vi "Locate Section.vi"(8 "error in":errorcluster, 10 "section":string, 11 "key lookup":variant) -> (0 "error out":errorcluster, 1 "Section Definition":T1, 2 "found?":bool, 3 "key lookup out":variant)   [LabVIEW 2012, in "configlib.lvlib"]
uses:
  configlib.lvlib
  Section Definition.ctl
  File Section.ctl
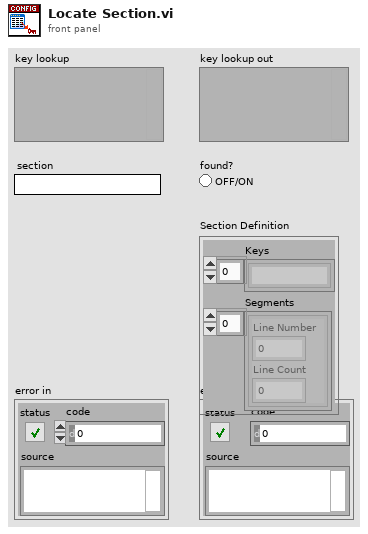
[diagram p1: front panel]
types:
  T1 = typedef "configlib.lvlib/Section Definition.ctl" = cluster{"Keys":string[], "Segments":T2[]}
  T2 = typedef "configlib.lvlib/File Section.ctl" = cluster{"Line Number":i32, "Line Count":i32}
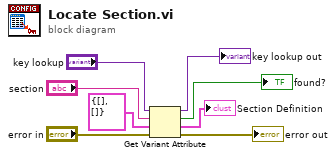
[diagram p0: block diagram]
diagram:
  n1 = Get Variant Attribute(Variant="key lookup", name="section", default value (empty Variant)=T1 {"Keys"=[], "Segments"=[]} ("Section Definition"), error in="error in") -> (duplicate Variant=→"key lookup out":variant, found=→"found?":bool, value=→"Section Definition":T1, error out=→"error out":errorcluster)
